vi "EvaluateHonor.vi"(10 "Count":u16[](array[numeric])) -> (1 "Pair":u16, 2 "Meld":u16)   [LabVIEW 2025]
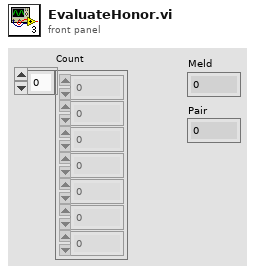
[diagram p1: front panel]
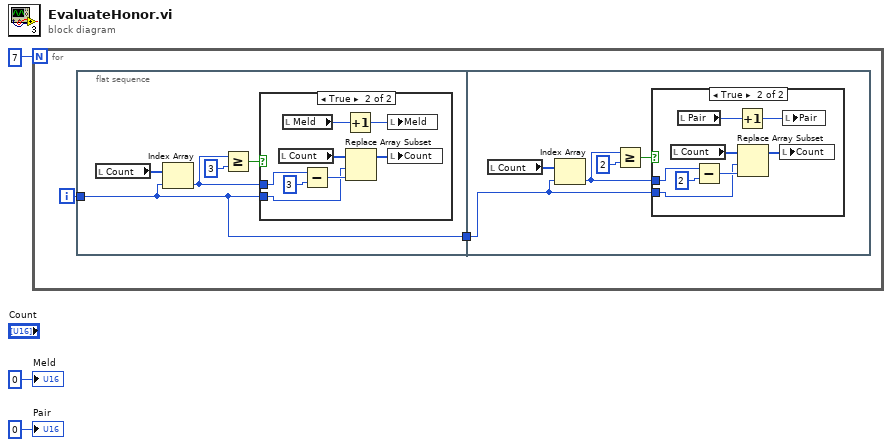
[diagram p0: block diagram]
diagram:
  n1 = for {
    N: 7 -> [_]
    i -> [w5]
    n2 = flat-sequence {
      tunnel: w5 -> [w6]
      tunnel: [w6] -> w4
      tunnel: w4 -> [w19]
      frame #0 {
        n3 = local read "Count"() -> (w10:u16[])
        n4 = Index Array(array=w10, index=w6) -> (element=w7:u16)
        n5 = Greater Or Equal?(x=w7, y=3) -> (x >= y?=w9:bool)
        n6 = case shown="True" w9 {
          tunnel: w7 -> [_ w13]
          tunnel: w6 -> [_ w11]
          frame False {
          }
          frame True {
            n7 = local read "Count"() -> (w15:u16[])
            n8 = local read "Meld"() -> (w18:u16)
            n9 = Subtract(x=w13, y=3) -> (x-y=w12:i32)
            n10 = Increment(x=w18) -> (x+1=w17:u16)
            n11 = Replace Array Subset(array=w15, new element=w12, index=w11) -> (w16:u16[])
            n12 = local write "Meld"(w17) -> ()
            n13 = local write "Count"(w16) -> ()
          }
        }
      }
      frame #1 {
        n14 = local read "Count"() -> (w20:u16[])
        n15 = Index Array(array=w20, index=w19) -> (element=w23:u16)
        n16 = Greater Or Equal?(x=w23, y=2) -> (x >= y?=w21:bool)
        n17 = case shown="True" w21 {
          tunnel: w23 -> [_ w26]
          tunnel: w19 -> [_ w24]
          frame False {
          }
          frame True {
            n18 = local read "Count"() -> (w28:u16[])
            n19 = local read "Pair"() -> (w31:u16)
            n20 = Subtract(x=w26, y=2) -> (x-y=w25:i32)
            n21 = Increment(x=w31) -> (x+1=w30:u16)
            n22 = Replace Array Subset(array=w28, new element=w25, index=w24) -> (w29:u16[])
            n23 = local write "Count"(w29) -> ()
            n24 = local write "Pair"(w30) -> ()
          }
        }
      }
    }
  }
  "Meld" <- u16 0 ("Meld")
  "Pair" <- u16 0 ("Pair")
